vi "Configure Active Step Of SEQ.vi"(8 "error in (no error)":errorcluster, 10 "SEQ step(1)":u8=1 min=1 max=10 step=1, 11 "VISA resource name":refnum<visa-resource-name>) -> (0 "error out":errorcluster, 3 "VISA resource name out":refnum<visa-resource-name>)   [LabVIEW 2020, in "IT6500.lvlib"]
doc: "This command is used to select the steps that the list sequence needs to be activated."
uses:
  IT6500.lvlib
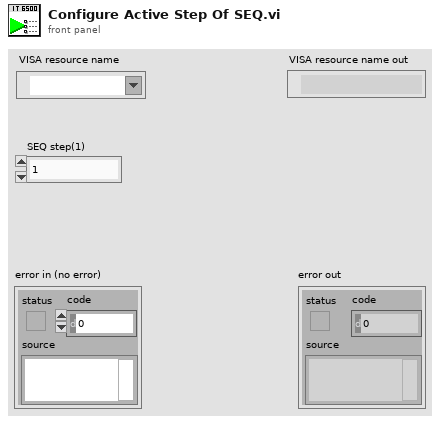
[diagram p1: front panel]
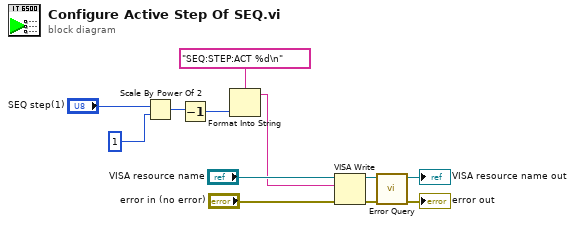
[diagram p0: block diagram]
diagram:
  n1 = Scale By Power Of 2(n="SEQ step(1)", x=1) -> (x*2^n=w4:i32)
  n2 = Decrement(x=w4) -> (x-1=w1:i32)
  n3 = Format Into String(format string="SEQ:STEP:ACT %d\n", w1) -> (resulting string=w6:string)  [unwired: 2 in, 1 out]
  n4 = VISA Write(VISA resource name="VISA resource name", write buffer=w6, error in (no error)="error in (no error)") -> (VISA resource name out=w9:refnum<visa-resource-name>, error out=w10:errorcluster)  [unwired: 1 out]
  n5 = call "Error Query.vi"("error in (no error)"=w10, "VISA resource name"=w9) -> ("error out"=→"error out":errorcluster, "VISA resource name out"=→"VISA resource name out":refnum<visa-resource-name>)  [unwired: 6 in, 2 out]
